vi "Create.vi"(9 "Actor":refnum<class "Actor.lvclass">, 10 "Self Alias":string, 11 "jettl Actor in":refnum<class "jettl Actor.lvclass">) -> (3 "jettl Actor out":refnum<class "jettl Actor.lvclass">)   [LabVIEW 2021, in "jettl.lvlib" / "Temporary Actor.lvlib" / "jettl Actor.lvclass"]
uses:
  jettl Actor.lvclass
  Actor/Actor.lvclass
  Init.ctl
  Msg/Msg.lvclass
  jettl Actor.lvclass/jettl Actor.ctl
  Addresses Strategy/Addresses Strategy/Addresses Strategy.lvclass
  Error/Error.lvlib
  C:/git/jettl/jettl/jettl/Temporary Actor/Actor/Actor.lvclass
  C:/git/jettl/jettl/jettl/Last Ack Msg/Last Ack/Last Ack.lvclass
  C:/git/jettl/jettl/jettl/Setup Msg/Setup/Setup.lvclass
  C:/git/jettl/jettl/jettl/Teardown Msg/Teardown/Teardown.lvclass
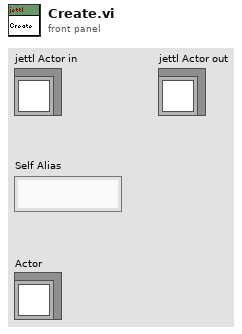
[diagram p1: front panel]
types:
  T1 = typedef "jettl.lvlib/Created Aliases.ctl" = set{string}
  T2 = typedef "jettl.lvlib/Temporary Actor.lvlib/jettl Actor.lvclass/Init.ctl" = cluster{"Self":refnum<user-event>, "Is Nominal State?":bool, "Temporary Flag":bool}
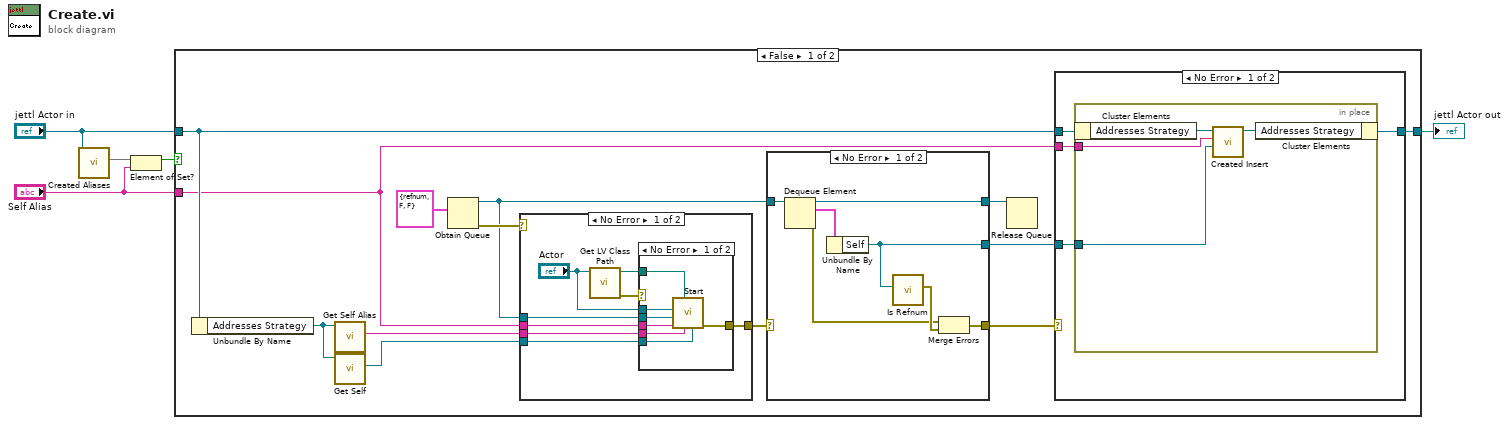
[diagram p0: block diagram]
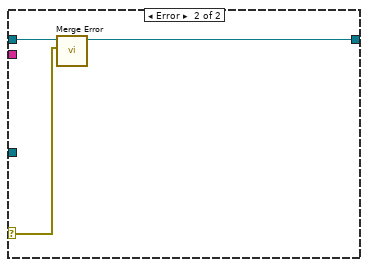
[diagram p5: hidden frame]
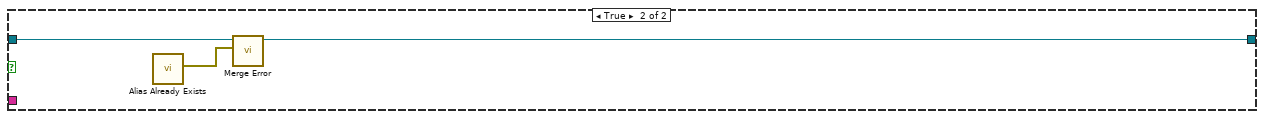
[diagram p6: hidden frame]
diagram:
  n1 = call-dynamic "Created Aliases.vi"("jettl Actor in"="jettl Actor in") -> ("Created Aliases"=w3:T1)  [unwired: 10 in]
  n2 = Element of Set?(10:"Self Alias", 11:w3) -> (3:w1:bool)
  n3 = case shown="False" w1 {
    tunnel: "jettl Actor in" -> [w14 w57]
    tunnel: "Self Alias" -> [w9 _]
    tunnel: [w18 w56] -> w5
    frame False {
      n4 = Unbundle By Name(w14) -> ("Addresses Strategy"=w13:refnum<class "Addresses Strategy.lvclass">)
      n5 = call-dynamic "Get Self Alias.vi"("Addresses Strategy in"=w13) -> ("Self Alias"=w11:string)  [unwired: 10 in]
      n6 = call-dynamic "Get Self.vi"("Addresses Strategy in"=w13) -> ("Self"=w12:refnum<user-event>)  [unwired: 10 in]
      n7 = Obtain Queue(element data type=T2 {"Self"=refnum, "Is Nominal State?"=FALSE, "Temporary Flag"=FALSE} ("Init")) -> (queue out=w10:refnum<queue>, error out=w17:errorcluster)  [unwired: 4 in, 1 out]
      n8 = case shown="No Error" w17 {
        selector: w17 -> [_ w44]
        tunnel: [w35 w44] -> w15
        tunnel: w9 -> [w32 _]
        tunnel: w12 -> [w34 _]
        tunnel: w11 -> [w33 _]
        tunnel: w10 -> [w31 _]
        frame No Error {
          n9 = call <vilib>:"Get LV Class Path.vi"("object"="Actor") -> ("error out"=w28:errorcluster, "class path"=w29:path)  [unwired: 9 in]
          n10 = case shown="No Error" w28 {
            selector: w28 -> [_ w43]
            tunnel: [w42 w43] -> w35
            tunnel: w34 -> [w41 _]
            tunnel: w33 -> [w40 _]
            tunnel: w32 -> [w39 _]
            tunnel: w31 -> [w36 _]
            tunnel: "Actor" -> [w38 _]
            tunnel: w29 -> [w37 _]
            frame No Error {
              n11 = call "Start.vi"("Creator"=w41, "Creator Alias"=w40, "Path"=w37, "Self Alias"=w39, "Queue of Init"=w36, "Actor"=w38) -> ("error out"=w42:errorcluster)  [unwired: 5 in]
            }
            frame Error {
            }
          }
        }
        frame Error {
        }
      }
      n12 = case shown="No Error" w15 {
        selector: w15 -> [_ w27]
        tunnel: [w25 w27] -> w16
        tunnel: w10 -> [w23 w26]
        tunnel: [w21 w26] -> w8
        tunnel: [w19 _] -> w6
        frame No Error {
          n13 = Dequeue Element(queue=w23) -> (queue out=w21:refnum<queue>, element=w20:T2, error out=w22:errorcluster)  [unwired: 2 in, 1 out]
          n14 = Unbundle By Name(w20) -> ("Self"=w19:refnum<user-event>)
          n15 = call "Is Refnum.vi"("Self"=w19) -> ("Error"=w24:errorcluster)  [unwired: 10 in]
          n16 = Merge Errors(w22, w24) -> (w25:errorcluster)
        }
        frame Error {
        }
      }
      n17 = Release Queue(queue=w8) -> ()  [unwired: 2 in, 3 out]
      n18 = case shown="No Error" w16 {
        selector: w16 -> [_ w55]
        tunnel: w14 -> [w47 w54]
        tunnel: [w46 w53] -> w18
        tunnel: w9 -> [w48 _]
        tunnel: w6 -> [w45 _]
        frame No Error {
          n19 = in-place {
            in-place-border: w48 -> [w50]
            in-place-border: w45 -> [w49]
            n20 = in-place-cluster #1(w47) -> ("Addresses Strategy"=w52:refnum<class "Addresses Strategy.lvclass">)
            n21 = call-dynamic "Created Insert.vi"("Created"=w49, "Created Alias"=w50, "Addresses Strategy in"=w52) -> ("Addresses Strategy out"=w51:refnum<class "Addresses Strategy.lvclass">)  [unwired: 8 in]
            n22 = in-place-cluster #1("Addresses Strategy"=w51) -> (w46:refnum<class "jettl Actor.lvclass">)
          }
        }
        frame Error {
          n23 = call-dynamic "Merge Error.vi"("Error"=w55, "jettl Actor in"=w54) -> ("jettl Actor out"=w53:refnum<class "jettl Actor.lvclass">)  [unwired: 9 in]
        }
      }
    }
    frame True {
      n24 = call "Alias Already Exists.vi"() -> ("Error"=w58:errorcluster)  [unwired: 11 in]
      n25 = call-dynamic "Merge Error.vi"("Error"=w58, "jettl Actor in"=w57) -> ("jettl Actor out"=w56:refnum<class "jettl Actor.lvclass">)  [unwired: 9 in]
    }
  }
  "jettl Actor out" <- w5
